vi "joystick.vi"() -> ()   [LabVIEW 2017]
uses:
  <vilib>/Utility/inputDevices.llb/closeKeyboard.vi
  <vilib>/Utility/inputDevices.llb/keyboardAcquire.vi
panel:
  out "Forward":bool
  out "A":bool
  out "Left":bool
  out "B":bool
  out "Back":bool
  out "X":bool
  out "Y":bool
  out "Right":bool
  out "update connection":bool
  in  "Power":dbl
  out "element":T1(ring)=enum."1"
  in  "stop":bool
  # "Cross (-1 - none; 0 - up; 90 - right; 180 - down; 270 - left)"
  # "Button:"
  # "Left stick"
  # "1 - A"
  # "2 - B"
  # "Triggers"
  # "3 - X"
  # "Right stick"
  # "4 - Y"
  # "5 - LB"
  # "6 - RB"
  # "7 - SELECT"
  # "8 - START"
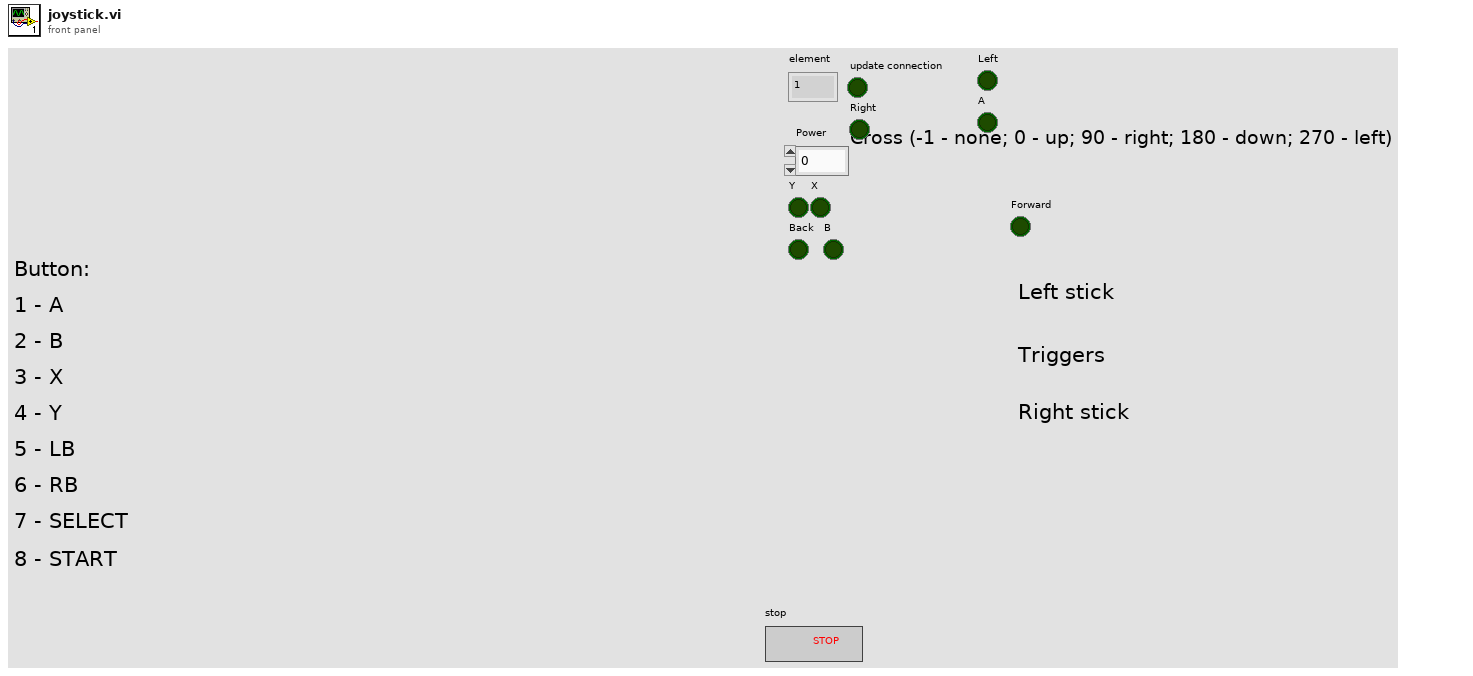
[diagram p1: front panel]
types:
  T1 = enum16{"0", "1", "2", "3", "4", "5", "6", "7", "8", "9", "A", "B", "C", "D", "E", "F", "G", "H", "I", "J", "K", "L", "M", "N", "O", "P", "Q", "R", "S", "T", "U", "V", "W", "X", "Y", "Z", "F1", "F2", "F3", "F4", "F5", "F6", "F7", "F8", "F9", "F10", "F11", "F12", "F13", "F14", "F15", "ADD", "BACK", "BACKSLASH", "CAPITAL", "COMMA", "DECIMAL", "DELETE", "DIVIDE", "DOWN", "END", "EQUALS", "ESCAPE", "GRAVE (`)", "HOME", "INSERT", "LBRACKET", "LCONTROL", "LEFT", "L ALT", "LSHIFT", "LWIN", "MINUS", "MULTIPLY", "NEXT", "NUMLOCK", "NUMPAD_0", "NUMPAD_1", "NUMPAD_2", "NUMPAD_3", "NUMPAD_4", "NUMPAD_5", "NUMPAD_6", "NUMPAD_7", "NUMPAD_8", "NUMPAD_9", "PAUSE", "PERIOD", "PRIOR (PG UP)", "RBRACKET", "RCONTROL", "RETURN", "RIGHT", "R ALT", "RSHIFT", "RWIN", "SCROLL", "SEMICOLON", "SLASH", "SPACE", "SUBTRACT", "TAB", "UP", "ENTER (num pad)", "' (quote)"}
  T2 = enum16{"0", "1", "2", "3", "4", "5", "6", "7", "8", "9", "A", "B", "C", "D", "E", "F", "G", "H", "I", "J", "K", "L", "M", "N", "O", "P", "Q", "R", "S", "T", "U", "V", "W", "X", "Y", "Z", "F1", "F2", "F3", "F4", "F5", "F6", "F7", "F8", "F9", "F10", "F11", "F12", "F13", "F14", "F15", "ADD", "BACK", "BACKSLASH", "CAPITAL", "COMMA", "DECIMAL", "DELETE", "DIVIDE", "DOWN", "END", "EQUALS", "ESCAPE", "GRAVE (`)", "HOME", "INSERT", "LBRACKET", "LCONTROL", "LEFT", "L ALT", "LSHIFT", "LWIN", "MINUS", "MULTIPLY", "NEXT", "NUMLOCK", "NUMPAD_0", "NUMPAD_1", "NUMPAD_2", "NUMPAD_3", "NUMPAD_4", "NUMPAD_5", "NUMPAD_6", "NUMPAD_7", "NUMPAD_8", "NUMPAD_9", "PAUSE", "PERIOD", "PRIOR (PG UP)", "RBRACKET", "RCONTROL", "RETURN", "RIGHT", "R ALT", "RSHIFT", "RWIN", "SCROLL", "SEMICOLON", "SLASH", "SPACE", "SUBTRACT", "TAB", "UP", "ENTER (num pad)", "' (quote)"}[]
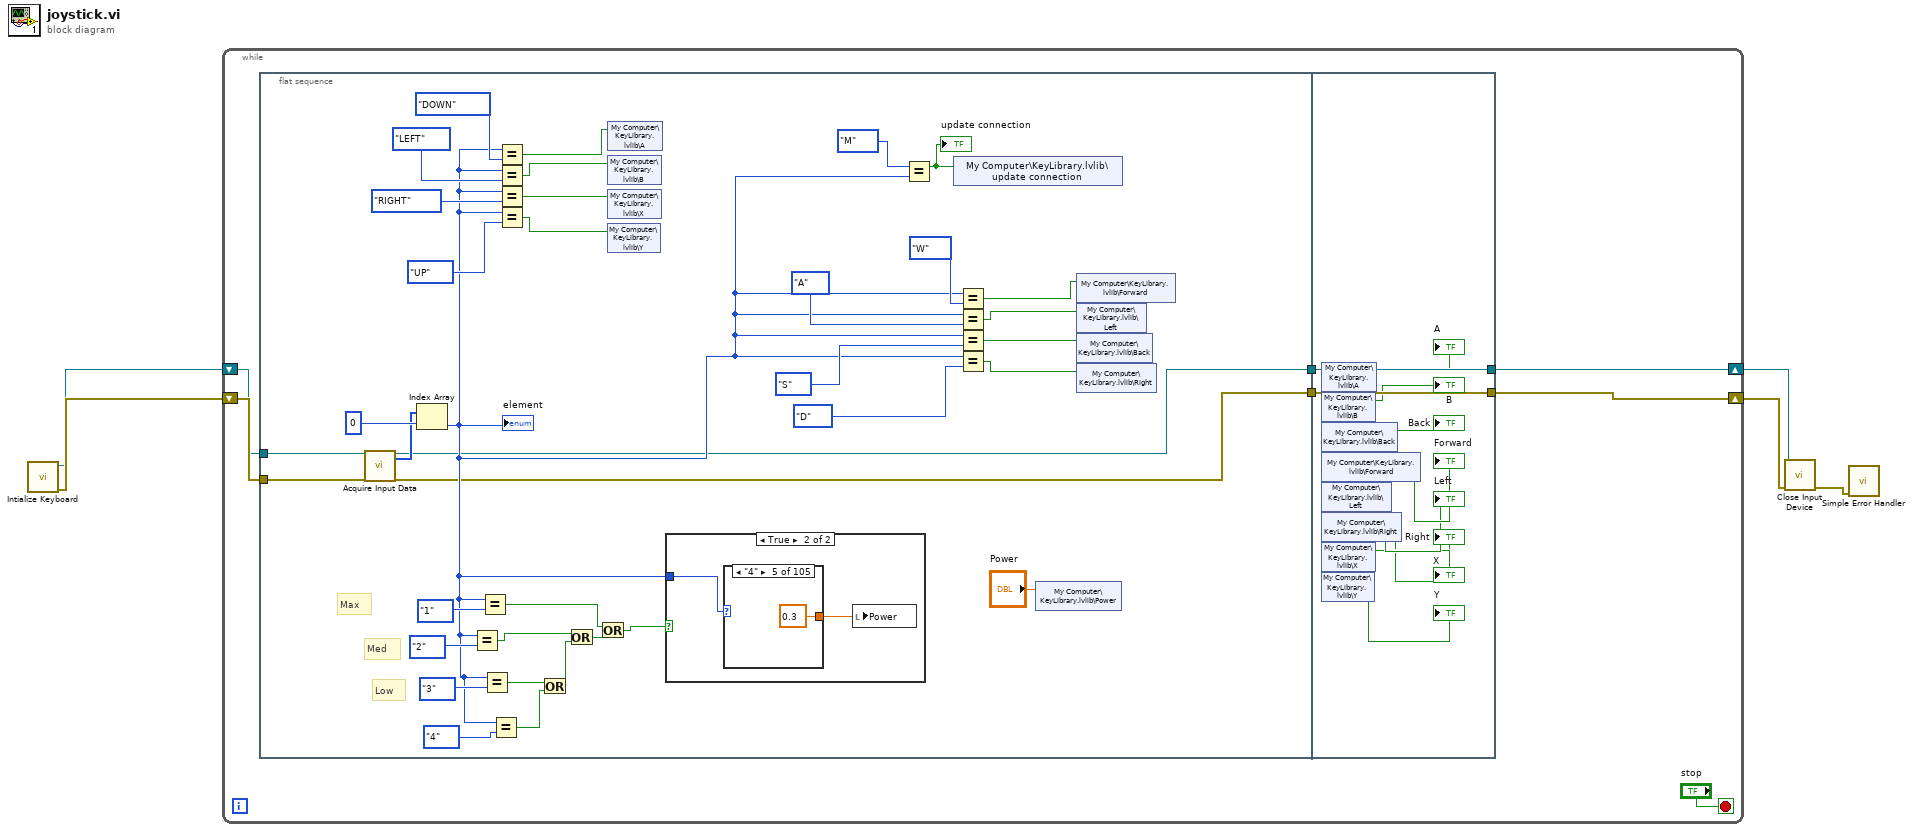
[diagram p0: block diagram]
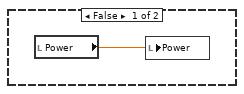
[diagram p2: hidden frame]
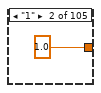
[diagram p4: hidden frame]
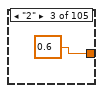
[diagram p5: hidden frame]
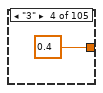
[diagram p6: hidden frame]
diagram:
  n1 = call <vilib>:"Intialize Keyboard.vi"() -> ("error out"=w2:errorcluster, "device ID"=w1:refnum<k1>)  [unwired: 10 in]
  n2 = while {
    shift-right: [w10] -> w4
    shift-left: w2 -> [w8]
    shift-right: [w9] -> w3
    shift-left: w1 -> [w7]
    stop <- "stop" stop-if-true
    n3 = flat-sequence {
      tunnel: w8 -> [w14]
      tunnel: w7 -> [w13]
      tunnel: [w16] -> w12
      tunnel: [w15] -> w11
      tunnel: [w65] -> w9
      tunnel: [w66] -> w10
      tunnel: w12 -> [w66]
      tunnel: w11 -> [w65]
      frame #0 {
        # "Low"
        # "Med"
        # "Max"
        n4 = call-poly <vilib>:"Acquire Input Data.vi"("device ID"=w13, "error in (no error)"=w14) -> ("device ID"=w15:refnum<k1>, "keys pressed"=w48:T2, "error out"=w16:errorcluster)  [unwired: 15 in]
        n5 = Index Array(array=w48, index=0 ("device index")) -> (element=w19:T1)
        "element" <- w19
        n6 = Equal?(x=w19, y=T1."2") -> (x = y?=w26:bool)
        n7 = Equal?(x=w19, y=T1."1") -> (x = y?=w27:bool)
        n8 = Equal?(x=w19, y=T1."3") -> (x = y?=w25:bool)
        n9 = Equal?(x=w19, y=T1."4") -> (x = y?=w20:bool)
        n10 = Equal?(x=w19, y=T1."DOWN") -> (x = y?=w43:bool)
        n11 = Equal?(x=w19, y=T1."LEFT") -> (x = y?=w42:bool)
        n12 = Equal?(x=w19, y=T1."RIGHT") -> (x = y?=w41:bool)
        n13 = Equal?(x=w19, y=T1."UP") -> (x = y?=w40:bool)
        n14 = Or(x=w25, y=w20) -> (x .or. y?=w21:bool)
        n15 = Or(x=w26, y=w21) -> (x .or. y?=w28:bool)
        n16 = Or(x=w27, y=w28) -> (x .or. y?=w24:bool)
        n17 = shared-variable "My Computer\\KeyLibrary.lvlib\\A"(w43) -> ()  [unwired: 1 in, 1 out]
        n18 = shared-variable "My Computer\\KeyLibrary.lvlib\\B"(w42) -> ()  [unwired: 1 in, 1 out]
        n19 = shared-variable "My Computer\\KeyLibrary.lvlib\\X"(w41) -> ()  [unwired: 1 in, 1 out]
        n20 = shared-variable "My Computer\\KeyLibrary.lvlib\\Y"(w40) -> ()  [unwired: 1 in, 1 out]
        n21 = case shown="True" w24 {
          tunnel: w19 -> [_ w52]
          frame False {
            n22 = local read "Power"() -> (w50:dbl)
            n23 = local write "Power"(w50) -> ()
          }
          frame True {
            n24 = case shown="\"4\"" w52 {
              tunnel: [_ 1.0 ("Power") 0.6 ("Power") 0.4 ("Power") 0.3 ("Power") _ _ _ _ _ _ _ _ _ _ _ _ _ _ _ _ _ _ _ _ _ _ _ _ _ _ _ _ _ _ _ _ _ _ _ _ _ _ _ _ _ _ _ _ _ _ _ _ _ _ _ _ _ _ _ _ _ _ _ _ _ _ _ _ _ _ _ _ _ _ _ _ _ _ _ _ _ _ _ _ _ _ _ _ _ _ _ _ _ _ _ _ _ _ _ _ _ _ _ _] -> w51
              frame "0", Default {
              }
              frame "1" {
              }
              frame "2" {
              }
              frame "3" {
              }
              frame "4" {
              }
              frame "5" {
              }
              frame "6" {
              }
              frame "7" {
              }
              frame "8" {
              }
              frame "9" {
              }
              frame "A" {
              }
              frame "B" {
              }
              frame "C" {
              }
              frame "D" {
              }
              frame "E" {
              }
              frame "F" {
              }
              frame "G" {
              }
              frame "H" {
              }
              frame "I" {
              }
              frame "J" {
              }
              frame "K" {
              }
              frame "L" {
              }
              frame "M" {
              }
              frame "N" {
              }
              frame "O" {
              }
              frame "P" {
              }
              frame "Q" {
              }
              frame "R" {
              }
              frame "S" {
              }
              frame "T" {
              }
              frame "U" {
              }
              frame "V" {
              }
              frame "W" {
              }
              frame "X" {
              }
              frame "Y" {
              }
              frame "Z" {
              }
              frame "F1" {
              }
              frame "F2" {
              }
              frame "F3" {
              }
              frame "F4" {
              }
              frame "F5" {
              }
              frame "F6" {
              }
              frame "F7" {
              }
              frame "F8" {
              }
              frame "F9" {
              }
              frame "F10" {
              }
              frame "F11" {
              }
              frame "F12" {
              }
              frame "F13" {
              }
              frame "F14" {
              }
              frame "F15" {
              }
              frame "ADD" {
              }
              frame "BACK" {
              }
              frame "BACKSLASH" {
              }
              frame "CAPITAL" {
              }
              frame "COMMA" {
              }
              frame "DECIMAL" {
              }
              frame "DELETE" {
              }
              frame "DIVIDE" {
              }
              frame "DOWN" {
              }
              frame "END" {
              }
              frame "EQUALS" {
              }
              frame "ESCAPE" {
              }
              frame "GRAVE (`)" {
              }
              frame "HOME" {
              }
              frame "INSERT" {
              }
              frame "LBRACKET" {
              }
              frame "LCONTROL" {
              }
              frame "LEFT" {
              }
              frame "L ALT" {
              }
              frame "LSHIFT" {
              }
              frame "LWIN" {
              }
              frame "MINUS" {
              }
              frame "MULTIPLY" {
              }
              frame "NEXT" {
              }
              frame "NUMLOCK" {
              }
              frame "NUMPAD_0" {
              }
              frame "NUMPAD_1" {
              }
              frame "NUMPAD_2" {
              }
              frame "NUMPAD_3" {
              }
              frame "NUMPAD_4" {
              }
              frame "NUMPAD_5" {
              }
              frame "NUMPAD_6" {
              }
              frame "NUMPAD_7" {
              }
              frame "NUMPAD_8" {
              }
              frame "NUMPAD_9" {
              }
              frame "PAUSE" {
              }
              frame "PERIOD" {
              }
              frame "PRIOR (PG UP)" {
              }
              frame "RBRACKET" {
              }
              frame "RCONTROL" {
              }
              frame "RETURN" {
              }
              frame "RIGHT" {
              }
              frame "R ALT" {
              }
              frame "RSHIFT" {
              }
              frame "RWIN" {
              }
              frame "SCROLL" {
              }
              frame "SEMICOLON" {
              }
              frame "SLASH" {
              }
              frame "SPACE" {
              }
              frame "SUBTRACT" {
              }
              frame "TAB" {
              }
              frame "UP" {
              }
              frame "ENTER (num pad)" {
              }
              frame "' (quote)" {
              }
            }
            n25 = local write "Power"(w51) -> ()
          }
        }
        n26 = Equal?(x=T1."M" ("y"), y=w19) -> (x = y?=w17:bool)
        "update connection" <- w17
        n27 = shared-variable "My Computer\\KeyLibrary.lvlib\\update connection"(w17) -> ()  [unwired: 1 in, 1 out]
        n28 = Equal?(x=w19, y=T1."W") -> (x = y?=w35:bool)
        n29 = Equal?(x=w19, y=T1."A") -> (x = y?=w34:bool)
        n30 = Equal?(x=w19, y=T1."S") -> (x = y?=w33:bool)
        n31 = Equal?(x=w19, y=T1."D") -> (x = y?=w32:bool)
        n32 = shared-variable "My Computer\\KeyLibrary.lvlib\\Power"("Power") -> ()  [unwired: 1 in, 1 out]
        n33 = shared-variable "My Computer\\KeyLibrary.lvlib\\Forward"(w35) -> ()  [unwired: 1 in, 1 out]
        n34 = shared-variable "My Computer\\KeyLibrary.lvlib\\Left"(w34) -> ()  [unwired: 1 in, 1 out]
        n35 = shared-variable "My Computer\\KeyLibrary.lvlib\\Back"(w33) -> ()  [unwired: 1 in, 1 out]
        n36 = shared-variable "My Computer\\KeyLibrary.lvlib\\Right"(w32) -> ()  [unwired: 1 in, 1 out]
      }
      frame #1 {
        n37 = shared-variable "My Computer\\KeyLibrary.lvlib\\A"() -> (→"A":bool)  [unwired: 1 in, 1 out]
        n38 = shared-variable "My Computer\\KeyLibrary.lvlib\\B"() -> (→"B":bool)  [unwired: 1 in, 1 out]
        n39 = shared-variable "My Computer\\KeyLibrary.lvlib\\Back"() -> (→"Back":bool)  [unwired: 1 in, 1 out]
        n40 = shared-variable "My Computer\\KeyLibrary.lvlib\\Forward"() -> (→"Forward":bool)  [unwired: 1 in, 1 out]
        n41 = shared-variable "My Computer\\KeyLibrary.lvlib\\Left"() -> (→"Left":bool)  [unwired: 1 in, 1 out]
        n42 = shared-variable "My Computer\\KeyLibrary.lvlib\\Right"() -> (→"Right":bool)  [unwired: 1 in, 1 out]
        n43 = shared-variable "My Computer\\KeyLibrary.lvlib\\X"() -> (→"X":bool)  [unwired: 1 in, 1 out]
        n44 = shared-variable "My Computer\\KeyLibrary.lvlib\\Y"() -> (→"Y":bool)  [unwired: 1 in, 1 out]
      }
    }
  }
  n45 = call-poly <vilib>:"Close Input Device.vi"("error in (no error)"=w4, "device ID"=w3) -> ("error out"=w5:errorcluster)  [unwired: 8 in]
  n46 = call <vilib>:"Simple Error Handler.vi"("error in (no error)"=w5) -> ()  [unwired: 4 in, 5 out]
